vi "Process.vi"(8 "error in (no error)":errorcluster, 10 "Initialize VPS in":refnum<class "Initialize VPS.lvclass">, 11 "Architecture.lvlib:Thread.lvclass":refnum<class "Thread.lvclass">) -> (0 "error out":errorcluster, 1 "Stop?":bool, 3 "Architecture.lvlib:Thread.lvclass 2":refnum<class "Thread.lvclass">)   [LabVIEW 2013, in "Vehicle Position Simulation.lvlib" / "Initialize VPS.lvclass"]
uses:
  Initialize VPS.lvclass
  Message.lvclass
  Thread.lvclass
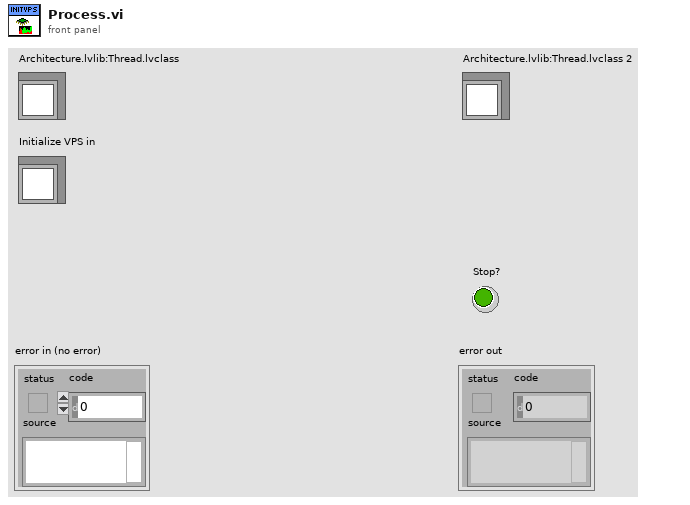
[diagram p1: front panel]
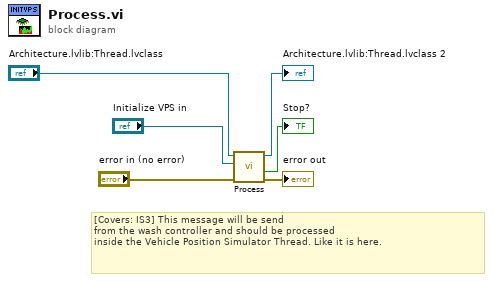
[diagram p0: block diagram]
diagram:
  # "[Covers: IS3] This message will be send\nfrom the wash controller and should be processed\ninside the Vehicle Position Simulator Thread. Like it is here."
  n1 = call-parent "Process.vi"("error in (no error)"="error in (no error)", "Message in"="Initialize VPS in", "Architecture.lvlib:Thread.lvclass"="Architecture.lvlib:Thread.lvclass") -> ("error out"=→"error out":errorcluster, "Stop?"=→"Stop?":bool, "Architecture.lvlib:Thread.lvclass 2"=→"Architecture.lvlib:Thread.lvclass 2":refnum<class "Thread.lvclass">)  [unwired: 6 in]
